vi "rsscope_core_global.vi"() -> ()   [LabVIEW 2018] (continued)
 Capabilities:\nNone\n\nRemote-control command(s):\nEXPort:WAVeform:SOURce"}, {"Level"=3, "Class Only"=FALSE, "Identifier"="RSSCOPE_ATTR_WAVEFORM_EXPORT_SCOPE", "Descriptive Name"="Waveform Export Scope", "Data Type"=0, "Command"="EXP:WAV:SCOP", "Access"=2, "Range Table"="rsscope_rngWaveformExportScope", "Read Callback"="", "Write Callback"="", "Supported Models"="", "Instrument Options"="", "Flags"=0, "Help"="Sets the part of the waveform record that has to be stored.\n\nAvailable Repeated Capabilities:\nNone\n\nRemote-control command(s):\nEXPort:WAVeform:SCOPe"}, {"Level"=3, "Class Only"=FALSE, "Identifier"="RSSCOPE_ATTR_WAVEFORM_EXPORT_SCOPE_CURSOR", "Descriptive Name"="Waveform Export Scope Cursor", "Data Type"=0, "Command"="EXP:WAV:CURS", "Access"=2, "Range Table"="rsscope_rngCursor", "Read Callback"="", "Write Callback"="", "Supported Models"="", "Instrument Options"="", "Flags"=0, "Help"="Sets the cursor set to be used for limited data export if RSSCOPE_ATTR_WAVEFORM_EXPORT_SCOPE is set to Cursor.\n\nAvailable Repeated Capabilities:\nNone\n\nRemote-control command(s):\nEXPort:WAVeform:CURSorset"}, {"Level"=3, "Class Only"=FALSE, "Identifier"="RSSCOPE_ATTR_WAVEFORM_EXPORT_SCOPE_GATE", "Descriptive Name"="Waveform Export Scope Gate", "Data Type"=0, "Command"="EXP:WAV:MEAS", "Access"=2, "Range Table"="rsscope_rngMeasurement", "Read Callback"="", "Write Callback"="", "Supported Models"="", "Instrument Options"="", "Flags"=0, "Help"="Sets the gate to be used for limited data export if RSSCOPE_ATTR_WAVEFORM_EXPORT_SCOPE is set to Gate.\n\nAvailable Repeated Capabilities:\nNone\n\nRemote-control command(s):\nEXPort:WAVeform:MEAS"}, {"Level"=3, "Class Only"=FALSE, "Identifier"="RSSCOPE_ATTR_WAVEFORM_EXPORT_SCOPE_START", "Descriptive Name"="Waveform Export Scope Start", "Data Type"=1, "Command"="EXP:WAV:STAR", "Access"=2, "Range Table"="rsscope_rngWaveformExportRange", "Read Callback"="", "Write Callback"="", "Supported Models"="", "Instrument Options"="", "Flags"=0, "Help"="Sets the start value of the waveform section for export, if RSSCOPE_ATTR_WAVEFORM_EXPORT_SCOPE is set to Manual.\n\nAvailable Repeated Capabilities:\nNone\n\nRemote-control command(s):\nEXPort:WAVeform:STARt"}, {"Level"=3, "Class Only"=FALSE, "Identifier"="RSSCOPE_ATTR_WAVEFORM_EXPORT_SCOPE_STOP", "Descriptive Name"="Waveform Export Scope Stop", "Data Type"=1, "Command"="EXP:WAV:STOP", "Access"=2, "Range Table"="rsscope_rngWaveformExportRange", "Read Callback"="", "Write Callback"="", "Supported Models"="", "Instrument Options"="", "Flags"=0, "Help"="Sets the end value of the waveform section for export, if RSSCOPE_ATTR_WAVEFORM_EXPORT_SCOPE is set to Manual.\n\nAvailable Repeated Capabilities:\nNone\n\nRemote-control command(s):\nEXPort:WAVeform:STOP"}, {"Level"=3, "Class Only"=FALSE, "Identifier"="RSSCOPE_ATTR_WAVEFORM_EXPORT_DATA_LOGGING", "Descriptive Name"="Waveform Export Data Logging", "Data Type"=3, "Command"="EXP:WAV:DLOG", "Access"=2, "Range Table"="", "Read Callback"="", "Write Callback"="", "Supported Models"="", "Instrument Options"="", "Flags"=0, "Help"="Enables the export of several subsequent waveforms into one file.\n\nAvailable Repeated Capabilities:\nNone\n\nRemote-control command(s):\nEXPort:WAVeform:DLOGging"}, {"Level"=3, "Class Only"=FALSE, "Identifier"="RSSCOPE_ATTR_WAVEFORM_EXPORT_TIMESTAMPS", "Descriptive Name"="Waveform Export Timestamps", "Data Type"=3, "Command"="EXP:WAV:TIM", "Access"=2, "Range Table"="", "Read Callback"="", "Write Callback"="", "Supported Models"="", "Instrument Options"="", "Flags"=0, "Help"="Exports the relative timestamps of all history waveforms to the waveform data file. The time is written at the beginning of each waveform record.\n\nAvailable Repeated Capabilities:\nNone\n\nRemote-control command(s):\nEXPort:WAVeform:TIMestamps"}, {"Level"=3, "Class Only"=FALSE, "Identifier"="RSSCOPE_ATTR_WAVEFORM_EXPORT_FAST_EXPORT", "Descriptive Name"="Waveform Export Fast Export", "Data Type"=3, "Command"="EXP:WAV:FAST", "Access"=1, "Range Table"="", "Read Callback"="", "Write Callback"="", "Supported Models"="", "Instrument Options"="", "Flags"=0, "Help"="To improve the performance of data export to file, the measurements are performed slower while the data export speeds up.\n\nAvailable Repeated Capabilities:\nNone\n\nRemote-control command(s):\nEXPort:WAVeform:FASTexport"}, {"Level"=3, "Class Only"=FALSE, "Identifier"="RSSCOPE_ATTR_WAVEFORM_EXPORT_FILE", "Descriptive Name"="Waveform Export File", "Data Type"=2, "Command"="EXP:WAV:NAME", "Access"=2, "Range Table"="", "Read Callback"="", "Write Callback"="", "Supported Models"="", "Instrument Options"="", "Flags"=0, "Help"="Stes the file name and path to save the waveform to.\n\nAvailable Repeated Capabilities:\nNone\n\nRemote-control command(s):\nEXPort:WAVeform:NAME"}, {"Level"=3, "Class Only"=FALSE, "Identifier"="RSSCOPE_ATTR_WAVEFORM_EXPORT", "Descriptive Name"="Waveform Export", "Data Type"=4, "Command"="EXP:WAV:SAVE", "Access"=1, "Range Table"="", "Read Callback"="", "Write Callback"="", "Supported Models"="", "Instrument Options"="", "Flags"=1, "Help"="Saves the waveform(s) to the file specified with RSSCOPE_ATTR_WAVEFORM_EXPORT_FILE.\n\nAvailable Repeated Capabilities:\nNone\n\nRemote-control command(s):\nEXPort:WAVeform:SAVE"}, {"Level"=3, "Class Only"=FALSE, "Identifier"="RSSCOPE_ATTR_WAVEFORM_EXPORT_INTERLEAVED_XY", "Descriptive Name"="Waveform Export Interleaved XY", "Data Type"=3, "Command"="EXP:WAV:INCX", "Access"=2, "Range Table"="", "Read Callback"="", "Write Callback"="", "Supported Models"="", "Instrument Options"="", "Flags"=0, "Help"="Includes horizontal values in the export data (time or frequency values, depending on the waveform). X and Y-values are written alternately to the file. If disabled, only Y-values - mostly voltage values - are written.\n\nAvailable Repeated Capabilities:\nNone\n\nRemote-control command(s):\nEXPort:WAVeform:INCXvalues"}, {"Level"=3, "Class Only"=FALSE, "Identifier"="RSSCOPE_ATTR_WAVEFORM_EXPORT_RAW_VALUES", "Descriptive Name"="Waveform Export Raw Values", "Data Type"=3, "Command"="EXP:WAV:RAW", "Access"=2, "Range Table"="", "Read Callback"="", "Write Callback"="", "Supported Models"="", "Instrument Options"="", "Flags"=0, "Help"="Enables the export of raw sample data of the ADC, and sets the data format to integer 8 bit. This format reduces the file size (1 Byte/sample instead of 4 Bytes/sample in binary files) but decreases the precision of the values.\n\nCurrently, the setting is not available for the export of digital channel data and for the export of interleaved X/Y values.\n\nAvailable Repeated Capabilities:\nNone\n\nRemote-control command(s):\nEXPort:WAVeform:RAW"}, {"Level"=3, "Class Only"=FALSE, "Identifier"="RSSCOPE_ATTR_WAVEFORM_EXPORT_DISPLAY_OFF", "Descriptive Name"="Waveform Export Display Off", "Data Type"=3, "Command"="EXP:WAV:DISP", "Access"=2, "Range Table"="", "Read Callback"="", "Write Callback"="", "Supported Models"="", "Instrument Options"="", "Flags"=0, "Help"="Enables or disables the display update during an Nx SINGLE acquisition.\n\nON: Disables the display update for maximum export speed.\nOFF: Enables the display update. The export is slower.\n\nAvailable Repeated Capabilities:\nNone\n\nRemote-control command(s):\nEXPort:WAVeform:DISPlayoff"}, {"Level"=3, "Class Only"=TRUE, "Identifier"="", "Descriptive Name"="Channel", "Data Type"=0, "Command"="", "Access"=0, "Range Table"="", "Read Callback"="", "Write Callback"="", "Supported Models"="", "Instrument Options"="", "Flags"=0, "Help"="This class attributes configures the storage settings for waveform data with channel repeated capability."}, {"Level"=4, "Class Only"=FALSE, "Identifier"="RSSCOPE_ATTR_WAVEFORM_EXPORT_CHANNEL", "Descriptive Name"="Waveform Export Channel", "Data Type"=3, "Command"="CHAN{Channel}:EXP", "Access"=2, "Range Table"="", "Read Callback"="", "Write Callback"="", "Supported Models"="", "Instrument Options"="", "Flags"=0, "Help"="Includes or excludes the indicated channel in waveform export. The data of channel waveform 1 is exported.\n\nAvailable Repeated Capabilities:\nChannel: CH1, CH2, CH3, CH4, CHExt\r\n\nRemote-control command(s):\nCHANnel<m>:EXPortstate"}, {"Level"=2, "Class Only"=TRUE, "Identifier"="", "Descriptive Name"="Histogram Export", "Data Type"=0, "Command"="", "Access"=0, "Range Table"="", "Read Callback"="", "Write Callback"="", "Supported Models"="", "Instrument Options"="", "Flags"=0, "Help"="This class attributes configures the storage settings for histogram waveform data."}, {"Level"=3, "Class Only"=FALSE, "Identifier"="RSSCOPE_ATTR_HISTOGRAM_EXPORT_NAME", "Descriptive Name"="Histogram Export Name", "Data Type"=2, "Command"="EXP:HIST:SEL", "Access"=2, "Range Table"="", "Read Callback"="", "Write Callback"="", "Supported Models"="", "Instrument Options"="", "Flags"=0, "Help"="Selects the histogram to be exported.\n\nAvailable Repeated Capabilities:\nNone\n\nRemote-control command(s):\nEXPort:HISTogram:SELect"}, {"Level"=3, "Class Only"=FALSE, "Identifier"="RSSCOPE_ATTR_HISTOGRAM_EXPORT_INCIDENCE", "Descriptive Name"="Histogram Export Incidence", "Data Type"=0, "Command"="EXP:HIST:INC", "Access"=2, "Range Table"="rsscope_rngAbsRel", "Read Callback"="", "Write Callback"="", "Supported Models"="", "Instrument Options"="", "Flags"=0, "Help"="Sets the mode of exported data: relative or absolute frequency of amplitude values\n\nAvailable Repeated Capabilities:\nNone\n\nRemote-control command(s):\nEXPort:HISTogram:INCidence"}, {"Level"=3, "Class Only"=FALSE, "Identifier"="RSSCOPE_ATTR_HISTOGRAM_EXPORT_FILE", "Descriptive Name"="Histogram Export File", "Data Type"=2, "Command"="EXP:HIST:NAME", "Access"=2, "Range Table"="", "Read Callback"="", "Write Callback"="", "Supported Models"="", "Instrument Options"="", "Flags"=0, "Help"="Stes the file name and path to save the histogram to.\n\nAvailable Repeated Capabilities:\nNone\n\nRemote-control command(s):\nEXPort:HISTogram:NAME"}, {"Level"=3, "Class Only"=FALSE, "Identifier"="RSSCOPE_ATTR_HISTOGRAM_EXPORT", "Descriptive Name"="Histogram Export", "Data Type"=4, "Command"="EXP:HIST:SAVE", "Access"=1, "Range Table"="", "Read Callback"="", "Write Callback"="", "Supported Models"="", "Instrument Options"="", "Flags"=1, "Help"="Saves the waveform(s) to the file specified with RSSCOPE_ATTR_HISTOGRAM_EXPORT_FILE.\n\nAvailable Repeated Capabilities:\nNone\n\nRemote-control command(s):\nEXPort:HISTogram:SAVE"}, {"Level"=2, "Class Only"=TRUE, "Identifier"="", "Descriptive Name"="Numeric Results", "Data Type"=0, "Command"="", "Access"=0, "Range Table"="", "Read Callback"="", "Write Callback"="", "Supported Models"="", "Instrument Options"="", "Flags"=0, "Help"="This class attributes configures the storage settings for numeric results."}, {"Level"=3, "Class Only"=FALSE, "Identifier"="RSSCOPE_ATTR_NUMERIC_RESULTS_DECIMAL_SYMBOL", "Descriptive Name"="Numeric Results Decimal Symbol", "Data Type"=0, "Command"="EXP:RES:DECS", "Access"=2, "Range Table"="RsScope_rngDecimalSymbol", "Read Callback"="", "Write Callback"="", "Supported Models"="", "Instrument Options"="", "Flags"=0, "Help"="Sets if point or comma is used as a decimal symbol.\n\nAvailable Repeated Capabilities:\nNone\n\nRemote-control command(s):\nEXPort:RESult:DECSymbol"}, {"Level"=3, "Class Only"=FALSE, "Identifier"="RSSCOPE_ATTR_NUMERIC_RESULTS_DELIMITER", "Descriptive Name"="Numeric Results Delimiter", "Data Type"=0, "Command"="EXP:RES:DEL", "Access"=2, "Range Table"="RsScope_rngDelimiter", "Read Callback"="", "Write Callback"="", "Supported Models"="", "Instrument Options"="", "Flags"=0, "Help"="Selects the value delimiter that is used to convert the values in columns. For MS Excel, the semicolon is recommended to be used.\n\nAvailable Repeated Capabilities:\nNone\n\nRemote-control command(s):\nEXPort:RESult:DELimiter"}, {"Level"=3, "Class Only"=FALSE, "Identifier"="RSSCOPE_ATTR_NUMERIC_RESULTS_OMIT_UNITS", "Descriptive Name"="Numeric Results Omit Units", "Data Type"=3, "Command"="EXP:RES:NUM", "Access"=2, "Range Table"="", "Read Callback"="", "Write Callback"="", "Supported Models"="", "Instrument Options"="", "Flags"=0, "Help"="If ON, the result values are saved without unit and with more decimal places.\n\nAvailable Repeated Capabilities:\nNone\n\nRemote-control command(s):\nEXPort:RESult:NUMeric"}, {"Level"=3, "Class Only"=FALSE, "Identifier"="RSSCOPE_ATTR_NUMERIC_RESULTS_EXPORT_FILE_NAME", "Descriptive Name"="Numeric Results Export File Name", "Data Type"=2, "Command"="EXP:RES:NAME", "Access"=2, "Range Table"="", "Read Callback"="", "Write Callback"="", "Supported Models"="", "Instrument Options"="", "Flags"=0, "Help"="Sets the path, the file name, and the file format for the numeric results file. Available file formats are CSV and HTML.\n\nAvailable Repeated Capabilities:\nNone\n\nRemote-control command(s):\nEXPort:RESult:NAME"}, {"Level"=3, "Class Only"=FALSE, "Identifier"="RSSCOPE_ATTR_NUMERIC_RESULTS_SAVE", "Descriptive Name"="Numeric Results Save", "Data Type"=4, "Command"="EXP:RES:SAVE", "Access"=1, "Range Table"="", "Read Callback"="", "Write Callback"="", "Supported Models"="", "Instrument Options"="", "Flags"=0, "Help"="Saves the selected result boxes to the file that is specified with RSSCOPE_ATTR_NUMERIC_RESULTS_EXPORT_FILE_NAME.\n\nAvailable Repeated Capabilities:\nNone\n\nRemote-control command(s):\nEXPort:RESult:SAVE"}, {"Level"=2, "Class Only"=TRUE, "Identifier"="", "Descriptive Name"="Long Term And Meas Histograms Export", "Data Type"=0, "Command"="", "Access"=0, "Range Table"="", "Read Callback"="", "Write Callback"="", "Supported Models"="", "Instrument Options"="", "Flags"=0, "Help"="This class attributes configures the storage settings for long term data."}, {"Level"=3, "Class Only"=FALSE, "Identifier"="RSSCOPE_ATTR_LONG_TERM_EXPORT_RESULT", "Descriptive Name"="Long Term Export Result", "Data Type"=0, "Command"="EXP:MEAS:SEL", "Access"=2, "Range Table"="rsscope_rngLongTermExportResult", "Read Callback"="", "Write Callback"="", "Supported Models"="", "Instrument Options"="", "Flags"=0, "Help"="This control selects the measurement to be exported.\n\nAvailable Repeated Capabilities:\nNone\n\nRemote-control command(s):\nEXPort:MEASurement:SELect"}, {"Level"=3, "Class Only"=FALSE, "Identifier"="RSSCOPE_ATTR_LONG_TERM_EXPORT_TYPE", "Descriptive Name"="Long Term Export Type", "Data Type"=0, "Command"="EXP:MEAS:TYPE", "Access"=2, "Range Table"="rsscope_rngLongTermExportType", "Read Callback"="", "Write Callback"="", "Supported Models"="", "Instrument Options"="", "Flags"=0, "Help"="Selects which result data you want to export, the long term Seasurement, or the measurement histogram.\n\nAvailable Repeated Capabilities:\nNone\n\nRemote-control command(s):\nEXPort:MEASurement:TYPE"}, {"Level"=3, "Class Only"=FALSE, "Identifier"="RSSCOPE_ATTR_LONG_TERM_EXPORT_FILE", "Descriptive Name"="Long Term Export File", "Data Type"=2, "Command"="EXP:MEAS:NAME", "Access"=2, "Range Table"="", "Read Callback"="", "Write Callback"="", "Supported Models"="", "Instrument Options"="", "Flags"=0, "Help"="Stes the file name and path to save the long term data.\n\nAvailable Repeated Capabilities:\nNone\n\nRemote-control command(s):\nEXPort:MEASurement:NAME"}, {"Level"=3, "Class Only"=FALSE, "Identifier"="RSSCOPE_ATTR_LONG_TERM_EXPORT", "Descriptive Name"="Long Term Export", "Data Type"=4, "Command"="EXP:MEAS:SAVE", "Access"=1, "Range Table"="", "Read Callback"="", "Write Callback"="", "Supported Models"="", "Instrument Options"="", "Flags"=1, "Help"="Saves the data to the file specified with RSSCOPE_ATTR_LONG_TERM_EXPORT_FILE\n\nAvailable Repeated Capabilities:\nNone\n\nRemote-control command(s):\nEXPort:MEASurement:SAVE"}, {"Level"=2, "Class Only"=TRUE, "Identifier"="", "Descriptive Name"="Reports", "Data Type"=0, "Command"="", "Access"=0, "Range Table"="", "Read Callback"="", "Write Callback"="", "Supported Models"="", "Instrument Options"="", "Flags"=0, "Help"="The following attributes configure and save report files."}, {"Level"=3, "Class Only"=FALSE, "Identifier"="RSSCOPE_ATTR_REPORT_LANGUAGE", "Descriptive Name"="Report Language", "Data Type"=2, "Command"="REP:LANG", "Access"=2, "Range Table"="", "Read Callback"="", "Write Callback"="", "Supported Models"="", "Instrument Options"="", "Flags"=0, "Help"="Selects the language to be used in the report. Available languages are listed in the data sheet.\n\nAvailable Repeated Capabilities:\nNone\n\nRemote-control command(s):\nREPort:LANGuage"}, {"Level"=3, "Class Only"=FALSE, "Identifier"="RSSCOPE_ATTR_REPORT_PAPER_SIZE", "Descriptive Name"="Report Paper Size", "Data Type"=0, "Command"="REP:PAP", "Access"=2, "Range Table"="RsScope_rngPowerAnalysisReportPaperSize", "Read Callback"="", "Write Callback"="", "Supported Models"="", "Instrument Options"="", "Flags"=0, "Help"="Selects the paper size: A4 or US Letter.\n\nAvailable Repeated Capabilities:\nNone\n\nRemote-control command(s):\nREPort:PAPersize"}, {"Level"=3, "Class Only"=FALSE, "Identifier"="RSSCOPE_ATTR_REPORT_USER", "Descriptive Name"="Report User", "Data Type"=2, "Command"="REP:USER", "Access"=2, "Range Table"="", "Read Callback"="", "Write Callback"="", "Supported Models"="", "Instrument Options"="", "Flags"=0, "Help"="Enter the user name that appears in the general information section at the beginning of the report.\n\nAvailable Repeated Capabilities:\nNone\n\nRemote-control command(s):\nREPort:USER"}, {"Level"=3, "Class Only"=FALSE, "Identifier"="RSSCOPE_ATTR_REPORT_COMMENT", "Descriptive Name"="Report Comment", "Data Type"=2, "Command"="REP:COMM", "Access"=2, "Range Table"="", "Read Callback"="", "Write Callback"="", "Supported Models"="", "Instrument Options"="", "Flags"=0, "Help"="Enter a comment that appears in the general information section at the beginning of the report.\n\nAvailable Repeated Capabilities:\nNone\n\nRemote-control command(s):\nREPort:COMMent"}, {"Level"=3, "Class Only"=FALSE, "Identifier"="RSSCOPE_ATTR_REPORT_LOGO_TYPE", "Descriptive Name"="Report Logo Type", "Data Type"=0, "Command"="REP:LOGT", "Access"=2, "Range Table"="RsScope_rngReportLogoType", "Read Callback"="", "Write Callback"="", "Supported Models"="", "Instrument Options"="", "Flags"=0, "Help"="By default, the Rohde & Schwarz logo is shown in the header of the report pages. You can switch the logo off, or select your logo to be shown.\n\nAvailable Repeated Capabilities:\nNone\n\nRemote-control command(s):\nREPort:LOGType"}, {"Level"=3, "Class Only"=FALSE, "Identifier"="RSSCOPE_ATTR_REPORT_LOGO_FILE", "Descriptive Name"="Report Logo File", "Data Type"=2, "Command"="REP:LOGO", "Access"=2, "Range Table"="", "Read Callback"="", "Write Callback"="", "Supported Models"="", "Instrument Options"="", "Flags"=0, "Help"="Defines the logo file that is used on the report if RSSCOPE_ATTR_REPORT_LOGO_TYPE is set to custom.\n\nAvailable Repeated Capabilities:\nNone\n\nRemote-control command(s):\nREPort:LOGO"}, {"Level"=3, "Class Only"=FALSE, "Identifier"="RSSCOPE_ATTR_REPORT_FILE_NAME", "Descriptive Name"="Report File Name", "Data Type"=2, "Command"="REP:FILE:NAME", "Access"=2, "Range Table"="", "Read Callback"="", "Write Callback"="", "Supported Models"="", "Instrument Options"="", "Flags"=0, "Help"="Sets the file name and path to save the report to. The file extension defines the file format: PDF, HTML, or DOC.\n\nAvailable Repeated Capabilities:\nNone\n\nRemote-control command(s):\nREPort:FILE:NAME"}, {"Level"=3, "Class Only"=FALSE, "Identifier"="RSSCOPE_ATTR_SAVE_REPORT", "Descriptive Name"="Save Report", "Data Type"=4, "Command"="REP:FILE:SAVE", "Access"=1, "Range Table"="", "Read Callback"="", "Write Callback"="", "Supported Models"="", "Instrument Options"="", "Flags"=0, "Help"="Saves the report to the specified file.\n\nAvailable Repeated Capabilities:\nNone\n\nRemote-control command(s):\nREPort:FILE:SAVE"}, {"Level"=2, "Class Only"=TRUE, "Identifier"="", "Descriptive Name"="Autonaming", "Data Type"=0, "Command"="", "Access"=0, "Range Table"="", "Read Callback"="", "Write Callback"="", "Supported Models"="", "Instrument Options"="", "Flags"=0, "Help"="In this tab you can define the pattern for automatic file name generation. This name is used as the default file name. The default path is the storage location for all saved files and their subdirectories."}, {"Level"=3, "Class Only"=FALSE, "Identifier"="RSSCOPE_ATTR_AUTONAMING_PREFIX", "Descriptive Name"="Autonaming Prefix", "Data Type"=3, "Command"="MMEM:AUT:PREF", "Access"=2, "Range Table"="", "Read Callback"="", "Write Callback"="", "Supported Models"="", "Instrument Options"="", "Flags"=0, "Help"="If enabled, inserts the default prefix in the file name. The prefix indicates the type of data that is saved, for example, Histogram, RefCurve, Settings.\n\nAvailable Repeated Capabilities:\nNone\n\nRemote-control command(s):\nMMEMory:AUTonaming:PREFix"}, {"Level"=3, "Class Only"=FALSE, "Identifier"="RSSCOPE_ATTR_AUTONAMING_TEXT", "Descriptive Name"="Autonaming Text", "Data Type"=2, "Command"="MMEM:AUT:TEXT", "Access"=2, "Range Table"="", "Read Callback"="", "Write Callback"="", "Supported Models"="", "Instrument Options"="", "Flags"=0, "Help"="User-defined text to be inserted after the prefix.\n\nAvailable Repeated Capabilities:\nNone\n\nRemote-control command(s):\nMMEMory:AUTonaming:TEXT"}, {"Level"=3, "Class Only"=FALSE, "Identifier"="RSSCOPE_ATTR_AUTONAMING_USER_TEXT", "Descriptive Name"="Autonaming User Text", "Data Type"=3, "Command"="MMEM:AUT:USER", "Access"=2, "Range Table"="", "Read Callback"="", "Write Callback"="", "Supported Models"="", "Instrument Options"="", "Flags"=0, "Help"="If enabled, inserts the specified user text after the prefix.\n\nAvailable Repeated Capabilities:\nNone\n\nRemote-control command(s):\nMMEMory:AUTonaming:USERtext"}, {"Level"=3, "Class Only"=FALSE, "Identifier"="RSSCOPE_ATTR_AUTONAMING_DATE", "Descriptive Name"="Autonaming Date", "Data Type"=3, "Command"="MMEM:AUT:DATE", "Access"=2, "Range Table"="", "Read Callback"="", "Write Callback"="", "Supported Models"="", "Instrument Options"="", "Flags"=0, "Help"="If enabled, inserts the current date.\n\nAvailable Repeated Capabilities:\nNone\n\nRemote-control command(s):\nMMEMory:AUTonaming:DATE"}, {"Level"=3, "Class Only"=FALSE, "Identifier"="RSSCOPE_ATTR_AUTONAMING_INDEX", "Descriptive Name"="Autonaming Index", "Data Type"=3, "Command"="MMEM:AUT:IND", "Access"=2, "Range Table"="", "Read Callback"="", "Write Callback"="", "Supported Models"="", "Instrument Options"="", "Flags"=0, "Help"="If enabled, inserts an index.\n\nAvailable Repeated Capabilities:\nNone\n\nRemote-control command(s):\nMMEMory:AUTonaming:INDex"}, {"Level"=3, "Class Only"=FALSE, "Identifier"="RSSCOPE_ATTR_AUTONAMING_TIME", "Descriptive Name"="Autonaming Time", "Data Type"=3, "Command"="MMEM:AUT:TIME", "Access"=2, "Range Table"="", "Read Callback"="", "Write Callback"="", "Supported Models"="", "Instrument Options"="", "Flags"=0, "Help"="If enabled, inserts the current time.\n\nAvailable Repeated Capabilities:\nNone\n\nRemote-control command(s):\nMMEMory:AUTonaming:TIME"}, {"Level"=3, "Class Only"=FALSE, "Identifier"="RSSCOPE_ATTR_AUTONAMING_DEFAULT_PATH", "Descriptive Name"="Autonaming Default Path", "Data Type"=2, "Command"="MMEM:AUT:DEF", "Access"=2, "Range Table"="", "Read Callback"="", "Write Callback"="", "Supported Models"="", "Instrument Options"="", "Flags"=0, "Help"="Defines the default path displayed in the file selection dialog box for loading and storing operations.\n\nAvailable Repeated Capabilities:\nNone\n\nRemote-control command(s):\nMMEMory:AUTonaming:DEFaultpath"}, {"Level"=3, "Class Only"=FALSE, "Identifier"="RSSCOPE_ATTR_AUTONAMING_RESET_PATH", "Descriptive Name"="Autonaming Reset Path", "Data Type"=4, "Command"="MMEM:AUT:RESP", "Access"=1, "Range Table"="", "Read Callback"="", "Write Callback"="", "Supported Models"="", "Instrument Options"="", "Flags"=0, "Help"="Resets the path for file operations to the default path.\n\nAvailable Repeated Capabilities:\nNone\n\nRemote-control command(s):\nMMEMory:AUTonaming:RESPath"}, {"Level"=3, "Class Only"=FALSE, "Identifier"="RSSCOPE_ATTR_AUTONAMING_RESET_ALL_SETTINGS", "Descriptive Name"="Autonaming Reset All Settings", "Data Type"=4, "Command"="MMEM:AUT:RES", "Access"=1, "Range Table"="", "Read Callback"="", "Write Callback"="", "Supported Models"="", "Instrument Options"="", "Flags"=0, "Help"="Resets all autonaming settings to the default value, including the path.\n\nAvailable Repeated Capabilities:\nNone\n\nRemote-control command(s):\nMMEMory:AUTonaming:RESall"}, {"Level"=1, "Class Only"=TRUE, "Identifier"="", "Descriptive Name"="Hardcopy and Printer", "Data Type"=0, "Command"="", "Access"=0, "Range Table"="", "Read Callback"="", "Write Callback"="", "Supported Models"="", "Instrument Options"="", "Flags"=0, "Help"="Configures Hardcopy and Printer."}, {"Level"=2, "Class Only"=FALSE, "Identifier"="RSSCOPE_ATTR_HARDCOPY_FILE_NAME", "Descriptive Name"="Hardcopy File Name", "Data Type"=2, "Command"="MMEM:NAME", "Access"=1, "Range Table"="", "Read Callback"="", "Write Callback"="", "Supported Models"="", "Instrument Options"="", "Flags"=0, "Help"="Defines the file name when an image of the display is stored to a file rather than printed to a printer using the HCOPy:IMMediate command.\n\nAvailable Repeated Capabilities:\nNone\n\nRemote-control command(s):\nMMEMory:NAME"}, {"Level"=2, "Class Only"=FALSE, "Identifier"="RSSCOPE_ATTR_HARDCOPY_PRINT", "Descriptive Name"="Hardcopy Print", "Data Type"=4, "Command"="HCOP:IMM", "Access"=1, "Range Table"="", "Read Callback"="", "Write Callback"="", "Supported Models"="", "Instrument Options"="", "Flags"=1, "Help"="Prints an image of the display to the printer or saves an image to a file or the clipboard, depending on the RSSCOPE_ATTR_HARDCOPY_DEVICE_DESTINATION attribute.\nThe printer is defined by RSSCOPE_ATTR_HARDCOPY_SELECT_PRINTER attribute. The file name for storage is defined by RSSCOPE_ATTR_HARDCOPY_FILE_NAME attribute.\n\nAvailable Repeated Capabilities:\nNone\n\nRemote-control command(s):\nHCOPy:IMMediate<m>[:DUM]"}, {"Level"=2, "Class Only"=FALSE, "Identifier"="RSSCOPE_ATTR_HARDCOPY_PRINT_NEXT", "Descriptive Name"="Hardcopy Print Next", "Data Type"=4, "Command"="HCOP:IMM:NEXT", "Access"=1, "Range Table"="", "Read Callback"="", "Write Callback"="", "Supported Models"="", "Instrument Options"="", "Flags"=0, "Help"="Starts the output of the next display image to printer, file, or clipboard, depending on the RSSCOPE_ATTR_HARDCOPY_DEVICE_DESTINATION attribute.\nIf the output is printed to a file, the file name used in the last saving process is automatically counted up to the next unused name.\n\nAvailable Repeated Capabilities:\nNone\n\nRemote-control command(s):\nHCOPy:IMMediate<m>:NEXT"}, {"Level"=2, "Class Only"=FALSE, "Identifier"="RSSCOPE_ATTR_HARDCOPY_GET_FIRST_PRINTER", "Descriptive Name"="Hardcopy Get First Printer", "Data Type"=2, "Command"="SYST:COMM:PRIN:ENUM:FIRS?", "Access"=0, "Range Table"="", "Read Callback"="", "Write Callback"="", "Supported Models"="", "Instrument Options"="", "Flags"=0, "Help"="This command queries the name of the first printer (in the list of printers) available under Windows XP.\n\nIf no printer is configured an empty string is output.\n\nAvailable Repeated Capabilities:\nNone\n\nRemote-control command(s):\nSYSTem:COMMunicate:PRINter:ENUMerate:FIRSt?"}, {"Level"=2, "Class Only"=FALSE, "Identifier"="RSSCOPE_ATTR_HARDCOPY_GET_NEXT_PRINTER", "Descriptive Name"="Hardcopy Get Next Printer", "Data Type"=2, "Command"="SYST:COMM:PRIN:ENUM:NEXT?", "Access"=0, "Range Table"="", "Read Callback"="", "Write Callback"="", "Supported Models"="", "Instrument Options"="", "Flags"=0, "Help"="This command queries the name of the next printer installed under Windows. After all available printer names have been output, an empty string enclosed by quotation marks (&apos;) is output for the next query. Further queries are answered by a query error.\nThe RSSCOPE_ATTR_HARDCOPY_GET_FIRST_PRINTER attribute should be sent previously to return to the beginning of the printer list and query the name of the first printer.\n\nAvailable Repeated Capabilities:\nNone\n\nRemote-control command(s):\nSYSTem:COMMunicate:PRINter:ENUMerate[:NEXT]?"}, {"Level"=2, "Class Only"=TRUE, "Identifier"="", "Descriptive Name"="Destination", "Data Type"=0, "Command"="", "Access"=0, "Range Table"="", "Read Callback"="", "Write Callback"="", "Supported Models"="", "Instrument Options"="", "Flags"=0, "Help"="Selects Destination."}, {"Level"=3, "Class Only"=FALSE, "Identifier"="RSSCOPE_ATTR_HARDCOPY_COLOR", "Descriptive Name"="Hardcopy Color", "Data Type"=3, "Command"="HCOP:DEV{Destination}:COL", "Access"=2, "Range Table"="", "Read Callback"="", "Write Callback"="", "Supported Models"="", "Instrument Options"="", "Flags"=0, "Help"="Defines the color mode for printing.\nON - color output\nOFF - black and white output\n\nAvailable Repeated Capabilities:\nDestination: DE1, DE2\r\n\nRemote-control command(s):\nHCOPy:DEVice<m>:COLor"}, {"Level"=3, "Class Only"=FALSE, "Identifier"="RSSCOPE_ATTR_HARDCOPY_DEVICE_DESTINATION", "Descriptive Name"="Hardcopy Device Destination", "Data Type"=0, "Command"="HCOP:DEST{Destination}", "Access"=2, "Range Table"="rsscope_rngHardcopyDevice", "Read Callback"="", "Write Callback"="rsscope_quotedInt_WriteCallback.vi", "Supported Models"="", "Instrument Options"="", "Flags"=0, "Help"="Selects the printer output medium (Disk, Printer or Clipboard).\n\nThe type of instrument is selected with SYSTem:COMMunicate:PRINter:SELect<1..2>, which automatically selects a default output medium. Therefore the HCOPy:DESTination command should always be sent after setting the device type.\n\nAvailable Repeated Capabilities:\nDestination: DE1, DE2\r\n\nRemote-control command(s):\nHCOPy:DESTination<1..2>"}, {"Level"=3, "Class Only"=FALSE, "Identifier"="RSSCOPE_ATTR_HARDCOPY_DEVICE_LANGUAGE_OUTPUT_FORMAT", "Descriptive Name"="Hardcopy Device Language Output Format", "Data Type"=0, "Command"="HCOP:DEV{Destination}:LANG", "Access"=2, "Range Table"="rsscope_rngHardcopyDeviceLang", "Read Callback"="", "Write Callback"="", "Supported Models"="", "Instrument Options"="", "Flags"=0, "Help"="Defines the file format for the image of the display.\n\nAvailable Repeated Capabilities:\nDestination: DE1, DE2\r\n\nRemote-control command(s):\nHCOPy:DEVice<m>:LANGuage"}, {"Level"=3, "Class Only"=FALSE, "Identifier"="RSSCOPE_ATTR_HARDCOPY_DEVICE_ORIENTATION", "Descriptive Name"="Hardcopy Device Orientation", "Data Type"=0, "Command"="HCOP:PAGE:ORI{Destination}", "Access"=2, "Range Table"="rsscope_rngHardcopyDeviceOrientation", "Read Callback"="", "Write Callback"="", "Supported Models"="", "Instrument Options"="", "Flags"=0, "Help"="Defines the page orientation.\n\nAvailable Repeated Capabilities:\nDestination: DE1, DE2\r\n\nRemote-control command(s):\nHCOPy:PAGE:ORIentation<1..2>"}, {"Level"=3, "Class Only"=FALSE, "Identifier"="RSSCOPE_ATTR_HARDCOPY_WHITE_BACKGROUND", "Descriptive Name"="Hardcopy White Background", "Data Type"=3, "Command"="HCOP:WBKG", "Access"=2, "Range Table"="", "Read Callback"="", "Write Callback"="", "Supported Models"="", "Instrument Options"="", "Flags"=0, "Help"="Inverts the background color. So you can print waveforms with normal waveform collors on white background.\n\nAvailable Repeated Capabilities:\nNone\n\nRemote-control command(s):\nHCOPy:WBKG"}, {"Level"=3, "Class Only"=FALSE, "Identifier"="RSSCOPE_ATTR_HARDCOPY_SELECT_PRINTER", "Descriptive Name"="Hardcopy Select Printer", "Data Type"=2, "Command"="SYST:COMM:PRIN:SEL{Destination}", "Access"=2, "Range Table"="", "Read Callback"="", "Write Callback"="", "Supported Models"="", "Instrument Options"="", "Flags"=0, "Help"="Selects a configured printer. To determine which printers are installed, use the RSSCOPE_ATTR_HARDCOPY_GET_FIRST_PRINTER and RSSCOPE_ATTR_HARDCOPY_GET_NEXT_PRINTER attributes.\n\nAvailable Repeated Capabilities:\nDestination: DE1, DE2\r\n\nRemote-control command(s):\nSYSTem:COMMunicate:PRINter:SELect<1..2>"}, {"Level"=3, "Class Only"=FALSE, "Identifier"="RSSCOPE_ATTR_HARDCOPY_PRINT_COLOR_SET", "Descriptive Name"="Hardcopy Print Color Set", "Data Type"=0, "Command"="HCOP:CMAP{Destination}:DEF", "Access"=2, "Range Table"="rsscope_rngHardcopyPrintColorSet", "Read Callback"="", "Write Callback"="", "Supported Models"="", "Instrument Options"="", "Flags"=0, "Help"="Defines the default color set for printing of the display image.\n\nAvailable Repeated Capabilities:\nDestination: DE1, DE2\r\n\nRemote-control command(s):\nHCOPy:CMAP<m>:DEFault"}, {"Level"=3, "Class Only"=FALSE, "Identifier"="RSSCOPE_ATTR_HARDCOPY_INVERSE_COLORS", "Descriptive Name"="Hardcopy Inverse Colors", "Data Type"=3, "Command"="HCOP:DEV{Destination}:INV", "Access"=2, "Range Table"="", "Read Callback"="", "Write Callback"="", "Supported Models"="", "Instrument Options"="", "Flags"=0, "Help"="Inverts the colors of the output, i.e. a dark waveform is printed on a white background.\n\nAvailable Repeated Capabilities:\nDestination: DE1, DE2\r\n\nRemote-control command(s):\nHCOPy:DEVice<m>:INVerse"}, {"Level"=3, "Class Only"=FALSE, "Identifier"="RSSCOPE_ATTR_HARDCOPY_INCLUDE_SIGNAL_BAR", "Descriptive Name"="Hardcopy Include Signal Bar", "Data Type"=3, "Command"="HCOP:ISBA", "Access"=2, "Range Table"="", "Read Callback"="", "Write Callback"="", "Supported Models"="", "Instrument Options"="", "Flags"=0, "Help"="If OFF, the screenshot shows only the diagram area, without the sidebar.\n\nAvailable Repeated Capabilities:\nNone\n\nRemote-control command(s):\nHCOPy:ISBA"}, {"Level"=3, "Class Only"=FALSE, "Identifier"="RSSCOPE_ATTR_HARDCOPY_SHOW_SETUP_DIALOG", "Descriptive Name"="Hardcopy Show Setup Dialog", "Data Type"=3, "Command"="HCOP:SSD", "Access"=2, "Range Table"="", "Read Callback"="", "Write Callback"="", "Supported Models"="", "Instrument Options"="", "Flags"=0, "Help"="Enables or disables the display of open dialog boxes in screenshots. Use this command if you want to document settings in screenshots.\n\nAvailable Repeated Capabilities:\nNone\n\nRemote-control command(s):\nHCOPy:SSD"}, {"Level"=1, "Class Only"=TRUE, "Identifier"="", "Descriptive Name"="External Application", "Data Type"=0, "Command"="", "Access"=0, "Range Table"="", "Read Callback"="", "Write Callback"="", "Supported Models"="", "Instrument Options"="", "Flags"=0, "Help"="Configure an external application that can be started at various events, for example, trigger event, or mask test violation."}, {"Level"=2, "Class Only"=FALSE, "Identifier"="RSSCOPE_ATTR_EXTERNAL_APPLICATION_NAME", "Descriptive Name"="External Application Name", "Data Type"=2, "Command"="EXEC:NAME", "Access"=2, "Range Table"="", "Read Callback"="", "Write Callback"="", "Supported Models"="", "Instrument Options"="", "Flags"=0, "Help"="Sets the path to the application executable.\n\nAvailable Repeated Capabilities:\nNone\n\nRemote-control command(s):\nEXECutable:NAME"}, {"Level"=2, "Class Only"=FALSE, "Identifier"="RSSCOPE_ATTR_EXTERNAL_APPLICATION_PARAMETER", "Descriptive Name"="External Application Parameter", "Data Type"=2, "Command"="EXEC:PAR", "Access"=2, "Range Table"="", "Read Callback"="", "Write Callback"="", "Supported Models"="", "Instrument Options"="", "Flags"=0, "Help"="Sets optional parameters for the external executable.\n\nAvailable Repeated Capabilities:\nNone\n\nRemote-control command(s):\nEXECutable:PARameter"}, {"Level"=2, "Class Only"=FALSE, "Identifier"="RSSCOPE_ATTR_EXTERNAL_APPLICATION_WORKING_DIRECTORY", "Descriptive Name"="External Application Working Directory", "Data Type"=2, "Command"="EXEC:WDIR", "Access"=2, "Range Table"="", "Read Callback"="", "Write Callback"="", "Supported Models"="", "Instrument Options"="", "Flags"=0, "Help"="Sets the working directory for the executable.\n\nAvailable Repeated Capabilities:\nNone\n\nRemote-control command(s):\nEXECutable:WDIRectory"}, {"Level"=1, "Class Only"=TRUE, "Identifier"="", "Descriptive Name"="Quick Action", "Data Type"=0, "Command"="", "Access"=0, "Range Table"="", "Read Callback"="", "Write Callback"="", "Supported Models"="", "Instrument Options"="", "Flags"=0, "Help"="Configures the Quick Action key on the instrument."}, {"Level"=2, "Class Only"=FALSE, "Identifier"="RSSCOPE_ATTR_QUICK_ACTION_MODE", "Descriptive Name"="Quick Action Mode", "Data Type"=0, "Command"="QACT:MODE", "Access"=2, "Range Table"="RsScope_rngQuickActionMode", "Read Callback"="", "Write Callback"="", "Supported Models"="", "Instrument Options"="", "Flags"=0, "Help"="Sets the action that is initiated by the Quick Action key.\n\nAvailable Repeated Capabilities:\nNone\n\nRemote-control command(s):\nQACTion:MODE"}, {"Level"=2, "Class Only"=FALSE, "Identifier"="RSSCOPE_ATTR_QUICK_ACTION_APPLICATION_PATH", "Descriptive Name"="Quick Action Application Path", "Data Type"=2, "Command"="QACT:PATH", "Access"=2, "Range Table"="", "Read Callback"="", "Write Callback"="", "Supported Models"="", "Instrument Options"="", "Flags"=0, "Help"="Sets the path to the application executable.\n\nAvailable Repeated Capabilities:\nNone\n\nRemote-control command(s):\nQACTion:PATH"}, {"Level"=2, "Class Only"=FALSE, "Identifier"="RSSCOPE_ATTR_QUICK_ACTION_PARAMETER", "Descriptive Name"="Quick Action Parameter", "Data Type"=2, "Command"="QACT:PAR", "Access"=2, "Range Table"="", "Read Callback"="", "Write Callback"="", "Supported Models"="", "Instrument Options"="", "Flags"=0, "Help"="Sets optional parameters for the external executable.\n\nAvailable Repeated Capabilities:\nNone\n\nRemote-control command(s):\nQACTion:PARameters"}, {"Level"=2, "Class Only"=FALSE, "Identifier"="RSSCOPE_ATTR_QUICK_ACTION_WORKING_DIRECTORY", "Descriptive Name"="Quick Action Working Directory", "Data Type"=2, "Command"="QACT:WDIR", "Access"=2, "Range Table"="", "Read Callback"="", "Write Callback"="", "Supported Models"="", "Instrument Options"="", "Flags"=0, "Help"="Sets the working directory for the executable.\n\nAvailable Repeated Capabilities:\nNone\n\nRemote-control command(s):\nQACTion:WDIRectory"}, {"Level"=2, "Class Only"=FALSE, "Identifier"="RSSCOPE_ATTR_QUICK_ACTION_EXECUTE", "Descriptive Name"="Quick Action Execute", "Data Type"=4, "Command"="QACT:EXEC", "Access"=1, "Range Table"="", "Read Callback"="", "Write Callback"="", "Supported Models"="", "Instrument Options"="", "Flags"=0, "Help"="Tests the Quick Action setup.\n\nAvailable Repeated Capabilities:\nNone\n\nRemote-control command(s):\nQACTion:EXECute"}, {"Level"=1, "Class Only"=TRUE, "Identifier"="", "Descriptive Name"="System", "Data Type"=0, "Command"="", "Access"=0, "Range Table"="", "Read Callback"="", "Write Callback"="", "Supported Models"="", "Instrument Options"="", "Flags"=0, "Help"="This class contains attributes that configure the system setup subsystem."}, {"Level"=2, "Class Only"=FALSE, "Identifier"="RSSCOPE_ATTR_CHANNEL_COUNT", "Descriptive Name"="Channel Count", "Data Type"=0, "Command"="DIAG:SERV:CHAN?", "Access"=0, "Range Table"="", "Read Callback"="", "Write Callback"="", "Supported Models"="", "Instrument Options"="", "Flags"=0, "Help"="Returns the channel count.\n\nAvailable Repeated Capabilities:\nNone\n\nRemote-control command(s):\nDIAGnostic:SERVice:CHANnelcount?"}, {"Level"=2, "Class Only"=FALSE, "Identifier"="RSSCOPE_ATTR_FIRMWARE_SHUTDOWN", "Descriptive Name"="Firmware Shutdown", "Data Type"=4, "Command"="SYST:EXIT", "Access"=1, "Range Table"="", "Read Callback"="", "Write Callback"="", "Supported Models"="", "Instrument Options"="", "Flags"=2, "Help"="Starts the shutdown of the firmware.\n\nAvailable Repeated Capabilities:\nNone\n\nRemote-control command(s):\nSYSTem:EXIT"}, {"Level"=2, "Class Only"=FALSE, "Identifier"="RSSCOPE_ATTR_FIRMWARE_VERSION", "Descriptive Name"="Firmware Version", "Data Type"=2, "Command"="DIAG:SERV:FWV?", "Access"=0, "Range Table"="", "Read Callback"="", "Write Callback"="", "Supported Models"="", "Instrument Options"="", "Flags"=0, "Help"="Returns 
